vi "LJUD_GetResultS.vi"(5 "Channel":i32, 7 "IOType":string, 8 "error in":errorcluster, 11 "Handle In":i32) -> (0 "error out":errorcluster, 2 "Value":dbl format="%.2f", 3 "Handle Out":i32)   [LabVIEW 2021]
doc: "In this version of GetResult the\nIOType is a string.\n\nGetResult is used to find the result\nassociated with a specific request\nirregardless of order.\n\nThis is a traditional technique UD\nfunction ... Add-Add-Go-Get-Get.\nSee Section 4.1 of the device's\ndatasheet for more information."
uses:
  labjackud.dll
panel:
  # "In this version of GetResult the\nIOType is a string.\n\nGetResult is used to find the result\nassociated with a specific request\nirregardless of order.\n\nThis is a traditional technique UD\nfunction ... Add-Add-Go-Get-Get.\nSee Section 4.1 of the device's\ndatasheet for more information."
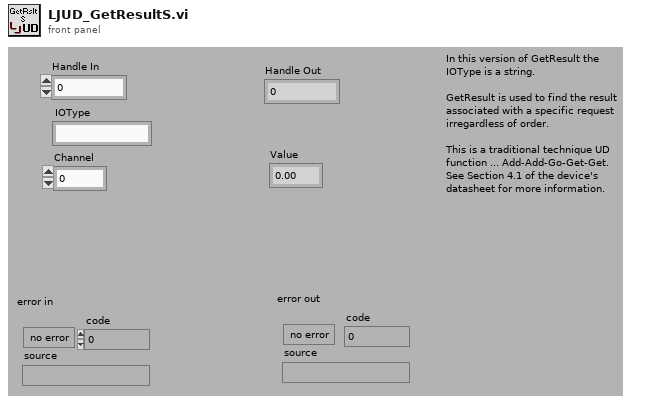
[diagram p1: front panel]
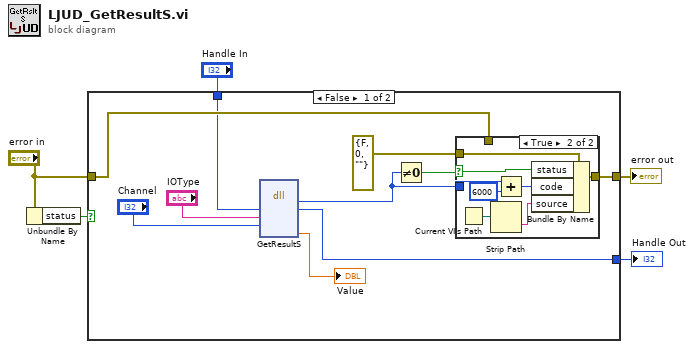
[diagram p0: block diagram]
diagram:
  n1 = Unbundle By Name("error in") -> ("status"=w4:bool)
  n2 = case shown="False" w4 {
    tunnel: [w9 w26] -> w5
    tunnel: "error in" -> [w8 w26]
    tunnel: "Handle In" -> [w7 w25]
    tunnel: [w6 w25] -> w1
    frame False {
      n3 = dll-call lib="labjackud.dll" fn="GetResultS"("Handle"=w7, "IOType"="IOType", "Channel"="Channel") -> (w11:i32, "Handle"=w6:i32, "Value"=→"Value":dbl)  [unwired: 6 in, 2 out]
      n4 = Not Equal To 0?(x=w11) -> (x != 0?=w10:bool)
      n5 = case shown="True" w10 {
        selector: w10 -> [_ w23]
        tunnel: [w16 w24] -> w9
        tunnel: errorcluster {"status"=FALSE, "code"=0, "source"=""} ("error IO") -> [_ w22]
        tunnel: w11 -> [_ w18]
        tunnel: w8 -> [w16 _]
        frame False {
        }
        frame True {
          n6 = Current VI's Path() -> (path=w20:path)
          n7 = Strip Path(path=w20) -> (name=w21:string)  [unwired: 1 out]
          n8 = Add(x=w18, y=6000) -> (x+y=w19:i32)
          n9 = Bundle By Name(cluster=w22, "status"=w23, "code"=w19, "source"=w21) -> (w24:errorcluster)
        }
      }
    }
    frame True {
    }
  }
  "error out" <- w5
  "Handle Out" <- w1
